vi "Actor Core.vi"(8 "error in":errorcluster, 11 "Error Log in":refnum<class "Error Log.lvclass">) -> (0 "error out":errorcluster, 3 "Actor out":refnum<class "Actor.lvclass">)   [LabVIEW 2023, in "Data Analysis.lvlib" / "Error Log.lvlib" / "Error Log.lvclass"]
doc: "(<B>Filename</B>: Actor Framework.lvlib:Actor.lvclass:Actor Core.vi)\n\nReceives messages to the actor, reacts to them, and initiates any error handling that may shut the actor down.\n\nDescendant classes may override this VI to append parallel tasks for the actor to complete while it handles messages. Overrides use the Call Parent Class Method node."
uses:
  Error Log.lvclass
  C:/Program Files/National Instruments/LabVIEW 2023/vi.lib/ActorFramework/Actor/Actor.lvclass
  <vilib>/ActorFramework/Actor/Actor.lvclass
  Error Log.lvclass/Error Log.ctl
  <vilib>/ActorFramework/Actor/Actor.lvclass/Actor.ctl
  <vilib>/ActorFramework/Message Enqueuer/Message Enqueuer.lvclass/Message Enqueuer.ctl
  Subpanel-Abstract Messages/Insert SP Msg/Insert SP Msg.lvclass/Insert SP Msg.ctl
  Error Log Messages/FE and FF Frame Error data Show Msg/FE and FF Frame Error data Show Msg.lvclass/FE and FF Frame Error data Show Msg.ctl
  <vilib>/ActorFramework/Message Enqueuer/Init from Existing Queue.vi
  <vilib>/ActorFramework/Message Enqueuer/Enqueue.vi
  Subpanel-Abstract Messages/Insert SP Msg/Insert SP Msg.lvclass
  C:/Program Files/National Instruments/LabVIEW 2023/vi.lib/ActorFramework/Message/Message.lvclass
  Error Log Messages/Initialise the Error log Based on Cycle number Msg/Initialise the Error log Based on Cycle number Msg.lvclass
  Error Log Messages/FE and FF Frame Error data Show Msg/FE and FF Frame Error data Show Msg.lvclass
  Error Log Messages/Error Tree Value Change and Cycle Numbers Msg/Error Tree Value Change and Cycle Numbers Msg.lvclass
  <vilib>/ActorFramework/Message Priority Queue/Priority Enqueue.vi
  <vilib>/ActorFramework/Message Enqueuer/Message Enqueuer.lvclass
  Subpanel-Abstract/Subpanel-Abstract.lvclass
  D:/eDCU LTT/VT LTT Project/Source Code/Data Analysis/Subpanel-Abstract/Subpanel-Abstract.lvclass
  D:/eDCU LTT/VT LTT Project/Source Code/Data Analysis/Error Log/Error Log/Error Log.lvclass
  Error Log Messages/Export Error Tree Data Msg/Export Error Tree Data Msg.lvclass
panel:
  in  "Save Button":bool
  in  "Cycle Filter":bool
  in  "Stop":bool
  in  "Error Data":i32(listbox)=-1 caption="Data"
  in  "Error_Tree":string(tree) caption="Error Log"
  # "Error Log"
  # "* Only Cycle Filters are applicable here"
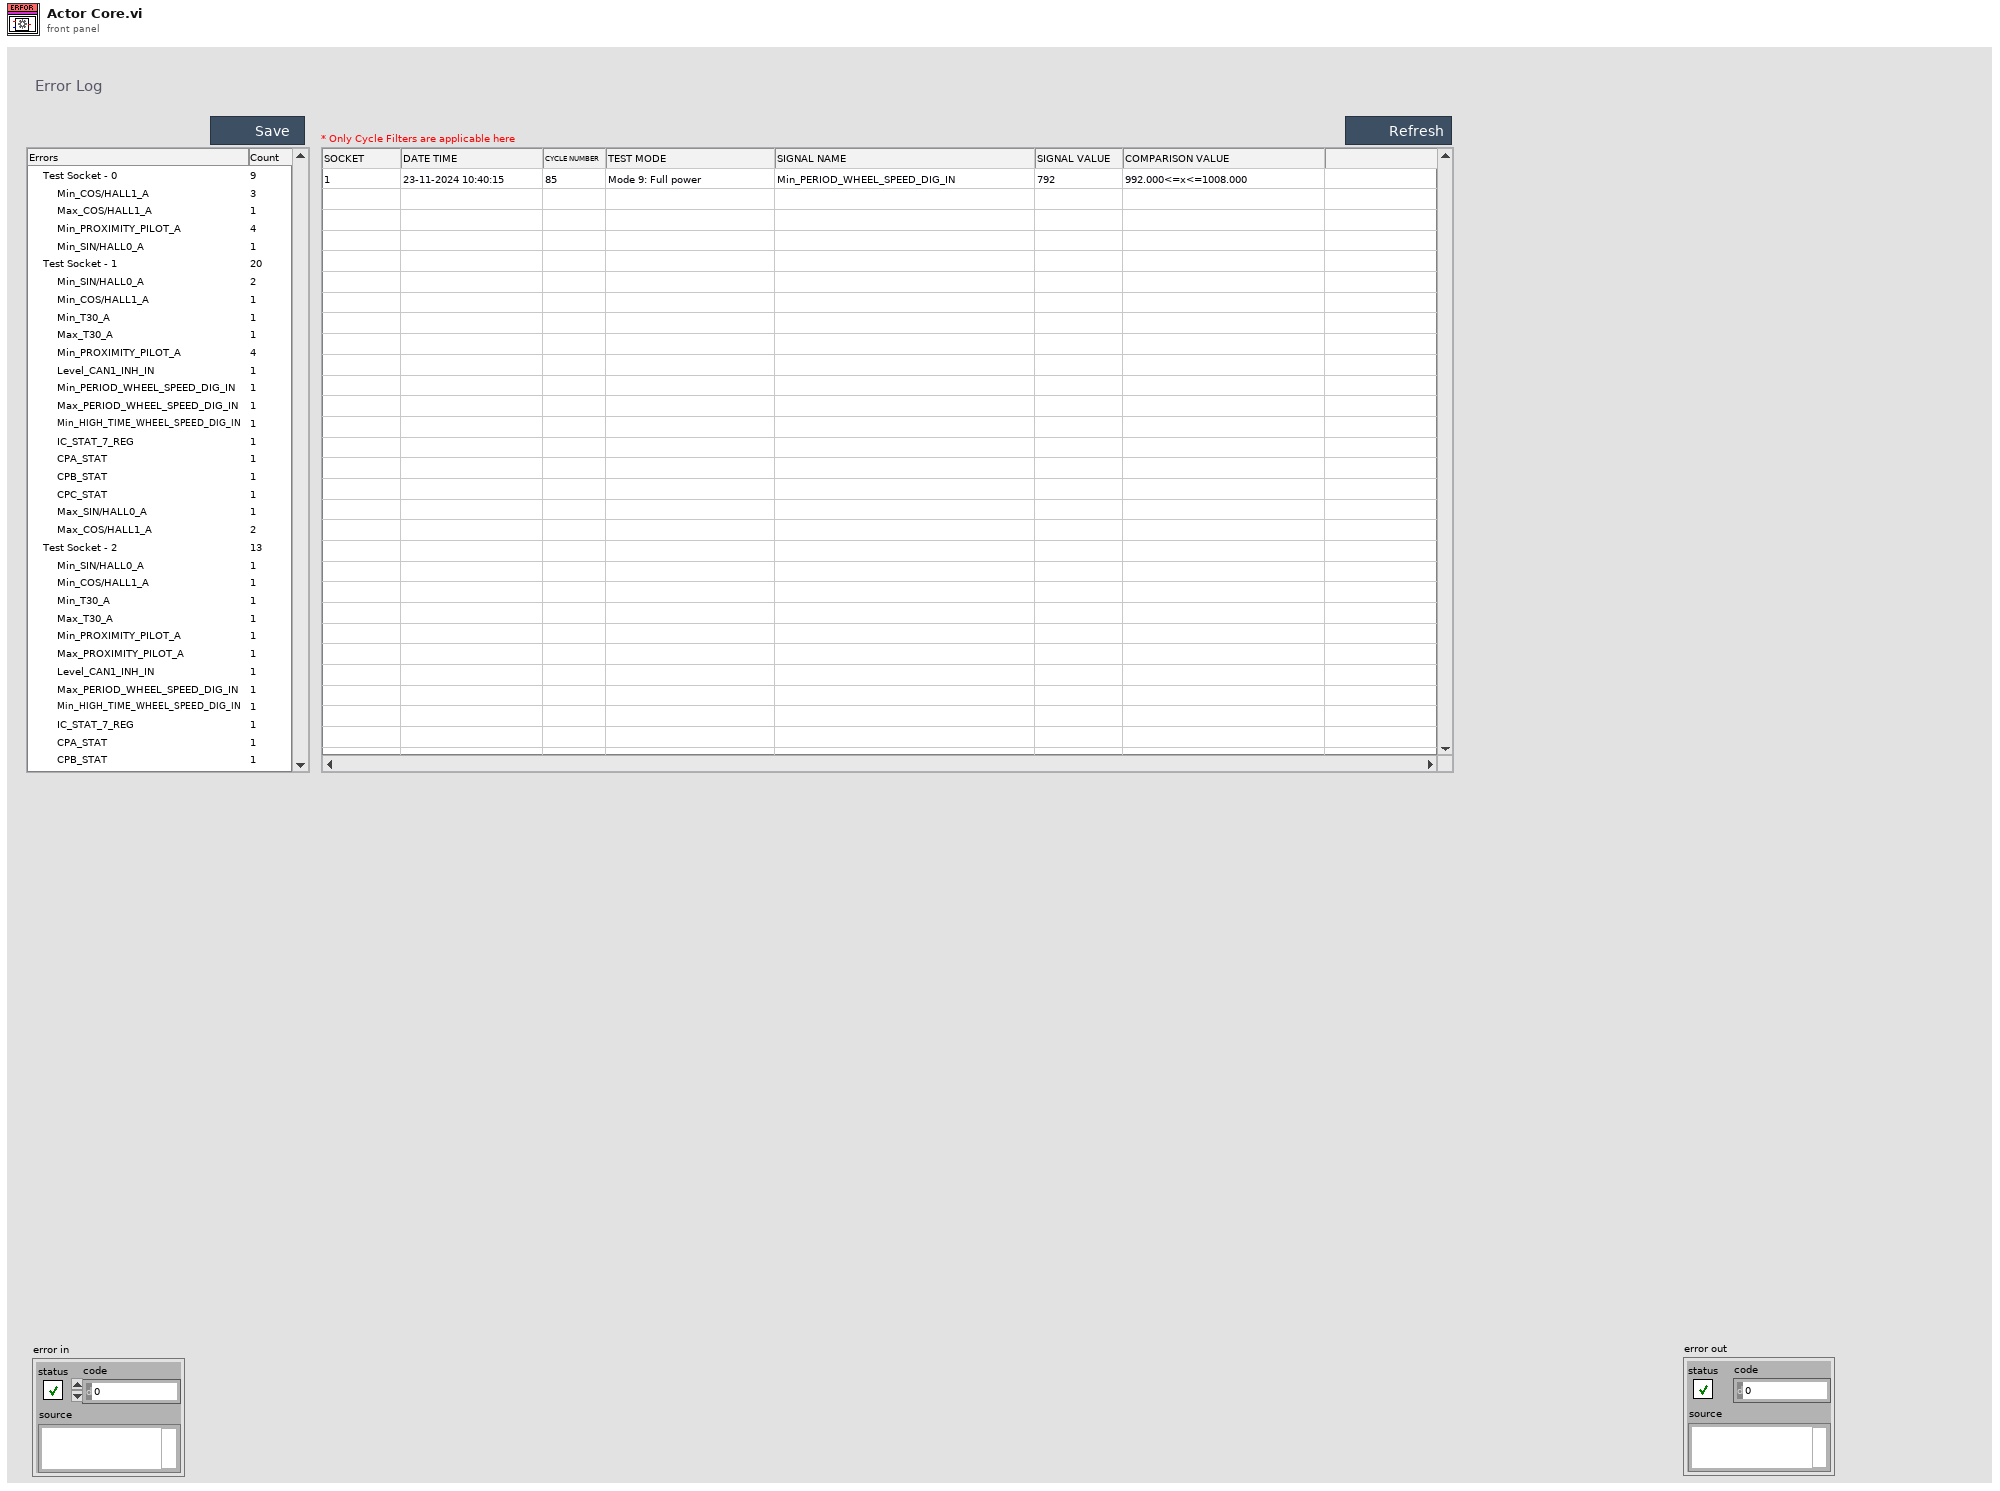
[diagram p1: front panel]
types:
  T1 = cluster{"Test Socket":string, "Test Cycle":string, "Test Mode":string}
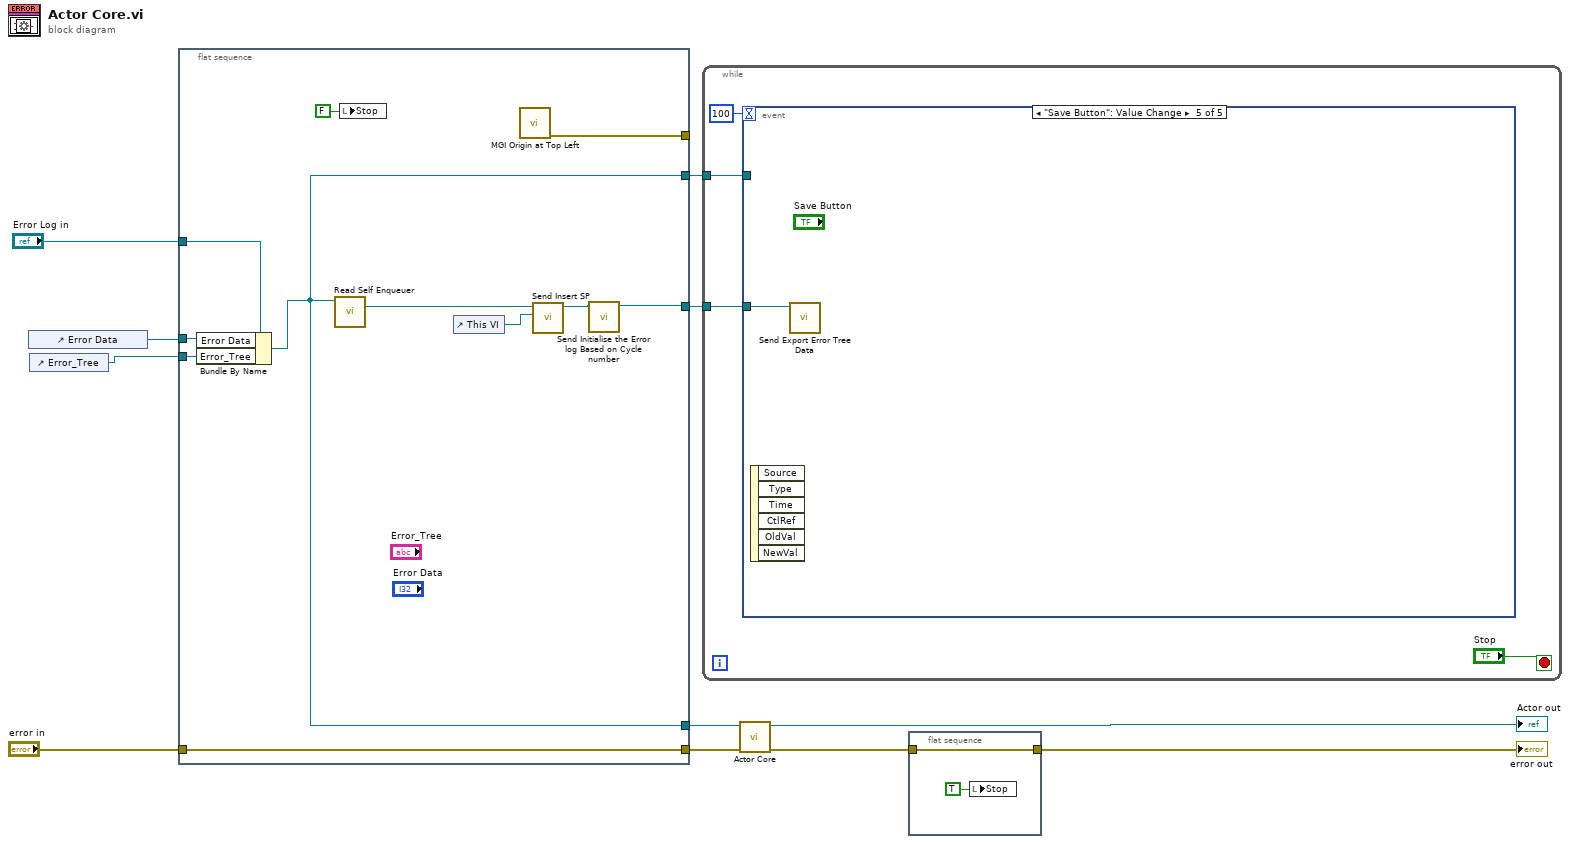
[diagram p0: block diagram]
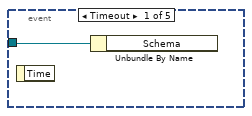
[diagram p2: hidden frame]
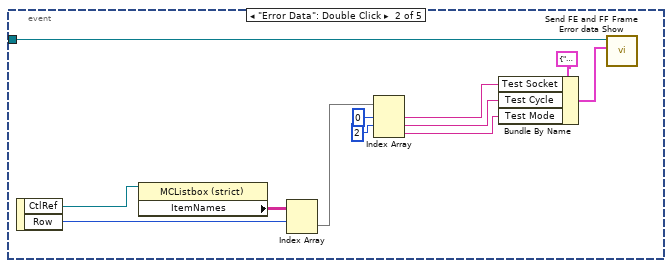
[diagram p3: hidden frame]
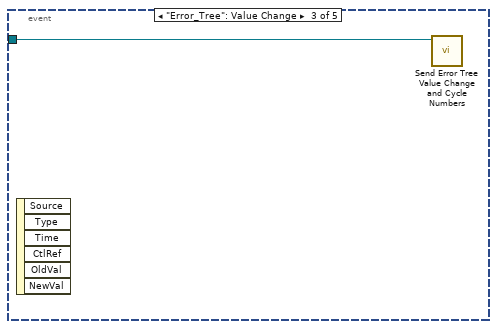
[diagram p4: hidden frame]
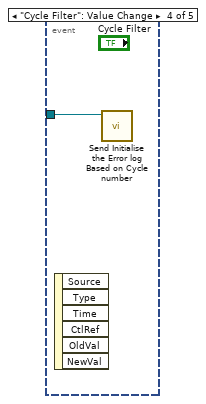
[diagram p5: hidden frame]
diagram:
  n1 = control-ref of="Error Data"() -> (w1:refnum<vi>)
  n2 = control-ref of="Error_Tree"() -> (w2:refnum<vi>)
  n3 = flat-sequence {
    tunnel: [w22] -> w9
    tunnel: "error in" -> [w22]
    tunnel: "Error Log in" -> [w18]
    tunnel: [w14] -> w7
    tunnel: [w12] -> w4
    tunnel: [w14] -> w3
    tunnel: [w19] -> _
    tunnel: w2 -> [w17]
    tunnel: w1 -> [w16]
    frame #0 {
      n4 = Bundle By Name(cluster=w18, "Error Data"=w16, "Error_Tree"=w17) -> (w14:refnum<class "Error Log.lvclass">)
      n5 = call <vilib>:"Read Self Enqueuer.vi"("Actor"=w14) -> ("Self Enqueuer"=w15:refnum<class "Message Enqueuer.lvclass">)  [unwired: 10 in]
      n6 = local write "Stop"(FALSE ("Stop")) -> ()
      n7 = control-ref of="This VI"() -> (w20:refnum<vi>)
      n8 = call <userlib>:"MGI Origin at Top Left.vi"() -> ("Error Out"=w19:errorcluster)  [unwired: 9 in, 1 out]
      n9 = call "Send Insert SP.vi"("VI Ref"=w20, "Message Enqueuer"=w15) -> ("Message Enqueuer out"=w13:refnum<class "Message Enqueuer.lvclass">)  [unwired: 8 in, 1 out]
      n10 = call "Send Initialise the Error log Based on Cycle number.vi"("Message Enqueuer"=w13) -> ("Message Enqueuer out"=w12:refnum<class "Message Enqueuer.lvclass">)  [unwired: 9 in, 1 out]
    }
  }
  n11 = while {
    tunnel: w4 -> [w24]
    tunnel: w3 -> [w23]
    stop <- "Stop" stop-if-true
    n12 = event shown="[4] \"Save Button\": Value Change" {
      selector: _ -> [_ _ _ _ _]
      dyn-events: _ -> [_ _ _ _ _]
      timeout: 100 -> [_ _ _ _ _]
      tunnel: w24 -> [_ w30 w40 w41 w42]
      tunnel: w23 -> [w27 _ _ _ _]
      event Timeout {
        n13 = event-data() -> ()  [unwired: 1 in, 1 out]
        n14 = Unbundle By Name(w27) -> ()  [unwired: 1 out]
      }
      event "Error Data": Double Click {
        n15 = event-data() -> ("CtlRef"=w31:refnum<vi>, "Row"=w32:i32)  [unwired: 1 in]
        n16 = property class="MCListbox (strict)"(reference=w31) -> ("ItemNames"=w39:string[][])  [unwired: 1 in, 2 out]
        n17 = Index Array(array=w39, index (row)=w32) -> (element=w38:string[])  [unwired: 1 in]
        n18 = Index Array(array=w38, index #1=0 ("index"), index #2=2 ("index")) -> (element #1=w35:string, element #2=w34:string, element #3=w33:string)  [unwired: 1 in]
        n19 = Bundle By Name(cluster=T1 {"Test Socket"="", "Test Cycle"="", "Test Mode"=""} ("Report Data"), "Test Socket"=w35, "Test Cycle"=w34, "Test Mode"=w33) -> (w28:T1)
        n20 = call "Send FE and FF Frame Error data Show.vi"("Report Data"=w28, "Message Enqueuer"=w30) -> ()  [unwired: 8 in, 2 out]
      }
      event "Error_Tree": Value Change {
        n21 = event-data() -> ()  [unwired: 1 in, 6 out]
        n22 = call "Send Error Tree Value Change and Cycle Numbers.vi"("Message Enqueuer"=w40) -> ()  [unwired: 9 in, 2 out]
      }
      event "Cycle Filter": Value Change {
        n23 = event-data() -> ()  [unwired: 1 in, 6 out]
        n24 = call "Send Initialise the Error log Based on Cycle number.vi"("Message Enqueuer"=w41) -> ()  [unwired: 9 in, 2 out]
      }
      event "Save Button": Value Change {
        n25 = event-data() -> ()  [unwired: 1 in, 6 out]
        n26 = call "Send Export Error Tree Data.vi"("Message Enqueuer"=w42) -> ()  [unwired: 9 in, 2 out]
      }
    }
  }
  n27 = call-parent "Actor Core.vi"("error in"=w9, "Actor in"=w7) -> ("error out"=w6:errorcluster, "Actor out"=→"Actor out":refnum<class "Actor.lvclass">)  [unwired: 8 in]
  n28 = flat-sequence {
    tunnel: w6 -> [w44]
    tunnel: [w44] -> w5
    frame #0 {
      n29 = local write "Stop"(TRUE ("Stop")) -> ()
    }
  }
  "error out" <- w5
